vi "PlaneFit.vi"(6 "Planing y/n?":bool, 7 "Reset Clicks":bool, 8 "Y PEN":dbl, 10 "Nano Z":dbl, 11 "Position":cluster{"X":dbl, "Y":dbl, "Zpen":dbl}) -> (2 "Plane Height (m)":dbl, 3 "Clicks":i32, 5 "Planing Done?":bool)   [LabVIEW 2017]
uses:
  Program Files/National Instruments/LabVIEW 2019/user.lib/HapticSTM/HapticSTM.lvlib
  GlobalClicksHeight.vi
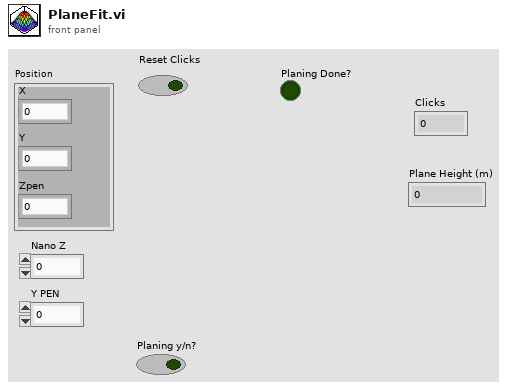
[diagram p1: front panel]
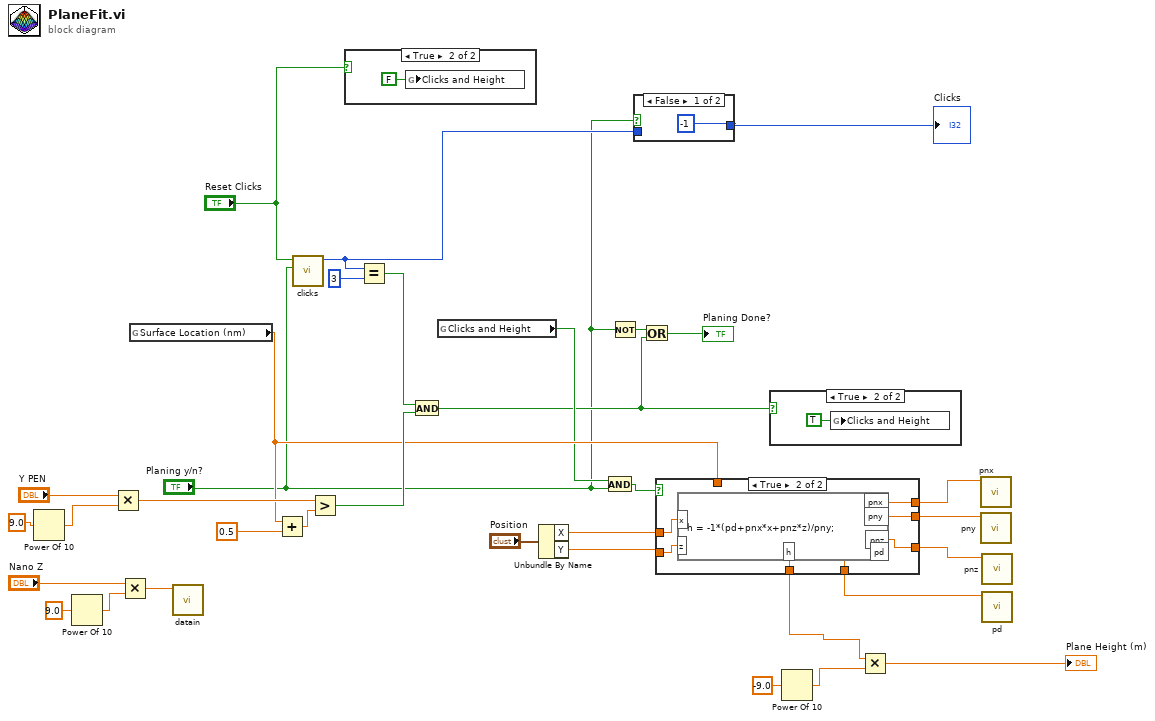
[diagram p0: block diagram]
diagram:
  n1 = Power Of 10(x=9.0) -> (10^x=w23:dbl)
  n2 = Power Of 10(x=9.0) -> (10^x=w19:dbl)
  n3 = Multiply(x="Y PEN", y=w23) -> (x*y=w20:dbl)
  n4 = Multiply(x="Nano Z", y=w19) -> (x*y=w15:dbl)
  n5 = global read "GlobalClicksHeight.vi" "Surface Location (nm)"() -> (w14:dbl)
  n6 = call "datain.vi"("output"=w15) -> ()  [unwired: 11 in]
  n7 = Add(x=w14, y=0.5) -> (x+y=w25:dbl)
  n8 = call "clicks.vi"("planing"="Planing y/n?", "reset"="Reset Clicks") -> ("function return"=w11:i32)  [unwired: 9 in]
  n9 = Greater?(x=w20, y=w25) -> (0:w26:bool)
  n10 = case shown="True" "Reset Clicks" {
    frame False {
    }
    frame True {
      n11 = global write "GlobalClicksHeight.vi" "Clicks and Height"(FALSE ("Clicks and Height")) -> ()
    }
  }
  n12 = Equal?(x=w11, y=3) -> (x = y?=w27:bool)
  n13 = And(x=w27, y=w26) -> (x .and. y?=w9:bool)
  n14 = global read "GlobalClicksHeight.vi" "Clicks and Height"() -> (w13:bool)
  n15 = Unbundle By Name("Position") -> ("X"=w2:dbl, "Y"=w1:dbl)
  n16 = And(x=w13, y="Planing y/n?") -> (x .and. y?=w12:bool)
  n17 = Not(x="Planing y/n?") -> (.not. x?=w7:bool)
  n18 = case shown="False" "Planing y/n?" {
    tunnel: w11 -> [_ w37]
    tunnel: [-1 ("function return") w37] -> w10
    frame False {
    }
    frame True {
    }
  }
  "Clicks" <- w10
  n19 = Or(x=w7, y=w9) -> (x .or. y?=→"Planing Done?":bool)
  n20 = case shown="True" w9 {
    frame False {
    }
    frame True {
      n21 = global write "GlobalClicksHeight.vi" "Clicks and Height"(TRUE ("Clicks and Height")) -> ()
    }
  }
  n22 = Power Of 10(x=-9.0) -> (10^x=w29:dbl)
  n23 = call "pnx.vi"() -> ("function return"=w31:dbl)  [unwired: 11 in]
  n24 = call "pny.vi"() -> ("function return"=w30:dbl)  [unwired: 11 in]
  n25 = call "pnz.vi"() -> ("function return"=w34:dbl)  [unwired: 11 in]
  n26 = call "pd.vi"() -> ("function return"=w33:dbl)  [unwired: 11 in]
  n27 = case shown="True" w12 {
    tunnel: w2 -> [_ w46]
    tunnel: w31 -> [_ w44]
    tunnel: w30 -> [_ w43]
    tunnel: w34 -> [_ w42]
    tunnel: w33 -> [_ w41]
    tunnel: w1 -> [_ w45]
    tunnel: [w39 w40] -> w4
    tunnel: w14 -> [w39 _]
    frame False {
    }
    frame True {
      n28 = formula code="h = -1*(pd+pnx*x+pnz*z)/pny;"("x"=w46, "z"=w45, "pnx"=w44, "pnz"=w42, "pd"=w41, "pny"=w43) -> ("h"=w40:dbl)
    }
  }
  n29 = Multiply(x=w4, y=w29) -> (x*y=→"Plane Height (m)":dbl)
